vi "Register gRPC Methods.vi"(8 "error in (no error)":errorcluster, 11 "Template Server in":refnum<class "Data Marshal Server.lvclass">) -> (0 "error out":errorcluster, 3 "Template Server out":refnum<class "Data Marshal Server.lvclass">)   [LabVIEW 2019, in "Data Marshal Server.lvlib" / "Data Marshal Server.lvclass"]
uses:
  Data Marshal Server.lvclass
  typeDefs/Server Internal UEs.ctl
  typeDefs/Server Internal Message.ctl
  typeDefs/Server gRPC UEs.ctl
  gRPC lvSupport/Server API/typeDefs/gRPCId Cluster.ctl
  gRPC lvSupport/Server API/typeDefs/grpcId.ctl
  Data Marshal Server.lvclass/Data Marshal Server.ctl
  gRPC lvSupport/gprc-lvsupport.lvlib
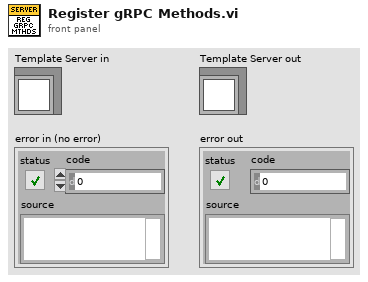
[diagram p1: front panel]
types:
  T1 = typedef "Data Marshal Server.lvlib/Data Marshal Server.lvclass/Server gRPC UEs.ctl" = cluster{"Invoke gRPC UE":refnum<user-event>, "Query gRPC UE":refnum<user-event>, "Register gRPC UE":refnum<user-event>, "TestDataTypes gRPC UE":refnum<user-event>}
  T2 = typedef "Data Marshal Server.lvlib/Data Marshal Server.lvclass/Server Internal UEs.ctl" = cluster{"Invoke Internal UE":refnum<user-event>, "Query Internal UE":refnum<user-event>, "Register Internal UE":refnum<user-event>, "TestDataTypes Internal UE":refnum<user-event>}
  T3 = typedef "Data Marshal Server.lvlib/gprc-lvsupport.lvlib/grpcId.ctl" = u64
  T4 = typedef "Data Marshal Server.lvlib/Data Marshal Server.lvclass/Server Internal Message UE.ctl" = refnum<user-event>
  T5 = typedef "Data Marshal Server.lvlib/gprc-lvsupport.lvlib/gRPCId Cluster UE.ctl" = refnum<user-event>
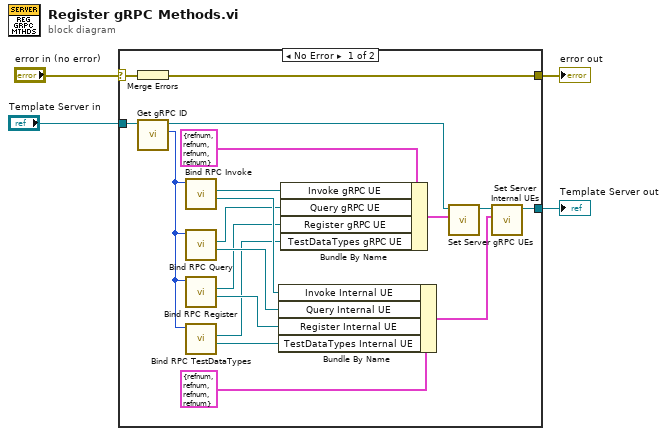
[diagram p0: block diagram]
diagram:
  n1 = case shown="No Error" "error in (no error)" {
    selector: "error in (no error)" -> [w14 w24]
    tunnel: "Template Server in" -> [w22 w25]
    tunnel: [w21 w24] -> w3
    tunnel: [w20 w25] -> w2
    frame No Error {
      n2 = Merge Errors(w14) -> (w21:errorcluster)
      n3 = call "Get gRPC ID.vi"("OOP Server in"=w22) -> ("gRPC ID"=w13:T3, "OOP Server out"=w23:refnum<class "Data Marshal Server.lvclass">)  [unwired: 9 in]
      n4 = call "Bind RPC Invoke.vi"("gRPCid server in"=w13) -> ("Invoke Internal UE"=w12:T4, "Invoke gRPC UE"=w11:T5)  [unwired: 7 in, 2 out]
      n5 = call "Bind RPC Query.vi"("gRPCid server in"=w13) -> ("Query Internal UE"=w10:T4, "Query gRPC UE"=w9:T5)  [unwired: 7 in, 2 out]
      n6 = call "Bind RPC Register.vi"("gRPCid server in"=w13) -> ("Register Internal UE"=w8:T4, "Register gRPC UE"=w7:T5)  [unwired: 7 in, 2 out]
      n7 = call "Bind RPC TestDataTypes.vi"("gRPCid server in"=w13) -> ("TestDataTypes Internal UE"=w6:T4, "TestDataTypes gRPC UE"=w5:T5)  [unwired: 7 in, 2 out]
      n8 = Bundle By Name ("Bundle Internal UEs")(cluster=T2 {"Invoke Internal UE"=refnum, "Query Internal UE"=refnum, "Register Internal UE"=refnum, "TestDataTypes Internal UE"=refnum} ("Server Internal UEs"), "Invoke Internal UE"=w12, "Query Internal UE"=w10, "Register Internal UE"=w8, "TestDataTypes Internal UE"=w6) -> (w19:T2)
      n9 = Bundle By Name ("Bundle gRPC UEs")(cluster=T1 {"Invoke gRPC UE"=refnum, "Query gRPC UE"=refnum, "Register gRPC UE"=refnum, "TestDataTypes gRPC UE"=refnum} ("gRPC Server Method Events"), "Invoke gRPC UE"=w11, "Query gRPC UE"=w9, "Register gRPC UE"=w7, "TestDataTypes gRPC UE"=w5) -> (w16:T1)
      n10 = call "Set Server gRPC UEs.vi"("Server gRPC UEs"=w16, "OOP Server in"=w23) -> ("OOP Server out"=w17:refnum<class "Data Marshal Server.lvclass">)  [unwired: 9 in]
      n11 = call "Set Server Internal UEs.vi"("Server Internal UEs"=w19, "OOP Server in"=w17) -> ("OOP Server out"=w20:refnum<class "Data Marshal Server.lvclass">)  [unwired: 9 in]
    }
    frame Error {
    }
  }
  "error out" <- w3
  "Template Server out" <- w2
